vi "ni579x Host Align.vi"(0 "sync.resources":T1, 1 "sync.meas.Reference Clock":refnum<k21>, 2 "sync.meas.FPGA Clock x2":refnum<k21>, 3 "sync.meas.FPGA I/O":refnum<k21>) -> (4 "sync.resources":T1)   [LabVIEW 2015, in "ni579x Synchronization v1 FPGA.lvlib"]
doc: "*** THIS VI IS DEPRECATED. USE ni579x Host Align 2.vi ***\n\nAlign the targets participating in synchronization. This must occur before a signal can be synchronized.\n\nThere are two flavors of alignment to chose from -- Host Align and FPGA Align. The two flavors produce the same quality of synchronization, but differ in requirements and versatility of operation.\n\nWhen using <B>ni579x FPGA Align 2</B>, the Single Cycle Timed Loop (SCTL) rate (that this VI is in) must be an integer multiple of the <B>sync.cptr.Reference Clock</B> rate, and the SCTL clock must have a fixed phase relationship to the reference clock. Each target performs its alignment independently, so FPGA Align does not require a FPGA I/O line. It's also possible to use FPGA Align without host interaction. FPGA Align has 100% repeatability if-and-only-if the target-to-target phase relationship is low and does not change.\n\nWhen using <B>ni579x Host Align 2</B>, the SCTL rate may be arbitrary (yet still must have a fixed phase relationship to the other targets). The CPTR period may also be arbitrary. This alignment process is coordinated by the host, and requires an FPGA I/O line for orchestration. Host Align has 100% repeatability; if the hardware configuration remains constant, so will the level of synchronization.\n\n<B>Input Parameters</B>\n\n<B>sync.resources</B> identifies the Synchronization instance. 'sync.resources' is obtained from the ni579x Create VI of this library.\n\n<B>sync.meas.Reference Clock</B> is used by the measurement logic as the \"start\" signal. This is commonly PXI_Clk10.\n\n<B>sync.meas.FPGA Clock x2</B> is used by the measurement logic as the measurement clock. This clock must run at twice the rate of the FPGA Clock (the clock that drives the Single Cycle Timed Loop (SCTL) which this VI is in). This clock must also be derrived from the FPGA Clock, so that it has a fixed phase relationship. This is commonly IO Module\\Sample Clock x2.\n\n<B>sync.meas.FPGA I/O</B> is the FPGA I/O line that will be used to orchestrate starting the measurements. This is commonly a PXI Trig line.\n\nNote: For large NI chassis, make sure the PXI Trig line is routed to all bus segments that have targets participating in synchronization.\n\n<B>Output Parameters</B>\n\n<B>sync.resources</B> is the same instance that was passed in for 'sync.resources'."
uses:
  <instrlib>/ni579x/Synchronization/v1/FPGA/ni579x Synchronization v1 FPGA.lvlib
  <vilib>/eio/EIONode/EIONode.xnode
  <instrlib>/_niInstr/Basic Elements/v1/FPGA/niInstr Basic Elements v1 FPGA.lvlib
  <vilib>/rvi/LocalResourceManager/LocalResourceManager.xnode
  <vilib>/rvi/DataTransferAndStorage/Container/Common/niFpgaContainerGetUniqueNameForEmu.vi
  <vilib>/rvi/DataTransferAndStorage/Container/Common/niFpgaContainerSetEmuInfo.vi
  <vilib>/rvi/eio/common/nirviEmuReportErrorAndStop.vi
  <instrlib>/_niInstr/TDC/v1/FPGA/niInstr Overclocked TDC v1 FPGA.lvlib
  <vilib>/rvi/eio/common/nirviEmuTemplateMethod_errors.vi
  <instrlib>/ni579x/Synchronization/v1/FPGA/Implementation/Resources.ctl
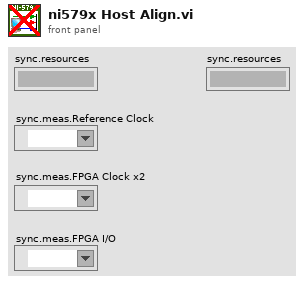
[diagram p1: front panel]
types:
  T1 = typedef "ni579x Synchronization v1 FPGA.lvlib/Resources.ctl" = cluster{"master":refnum<k21>, "meas.enable":refnum<k21>, "meas.ready":refnum<k21>, "meas.arm":refnum<k21>, "meas.valid":refnum<k21>, "meas.value":refnum<k21>, "meas.oversample clock":refnum<k21>, "meas.oversample factor":refnum<k21>, "cptr":refnum<k21>, "cptr.adjust":refnum<k21>, "cptr.period":refnum<k21>}
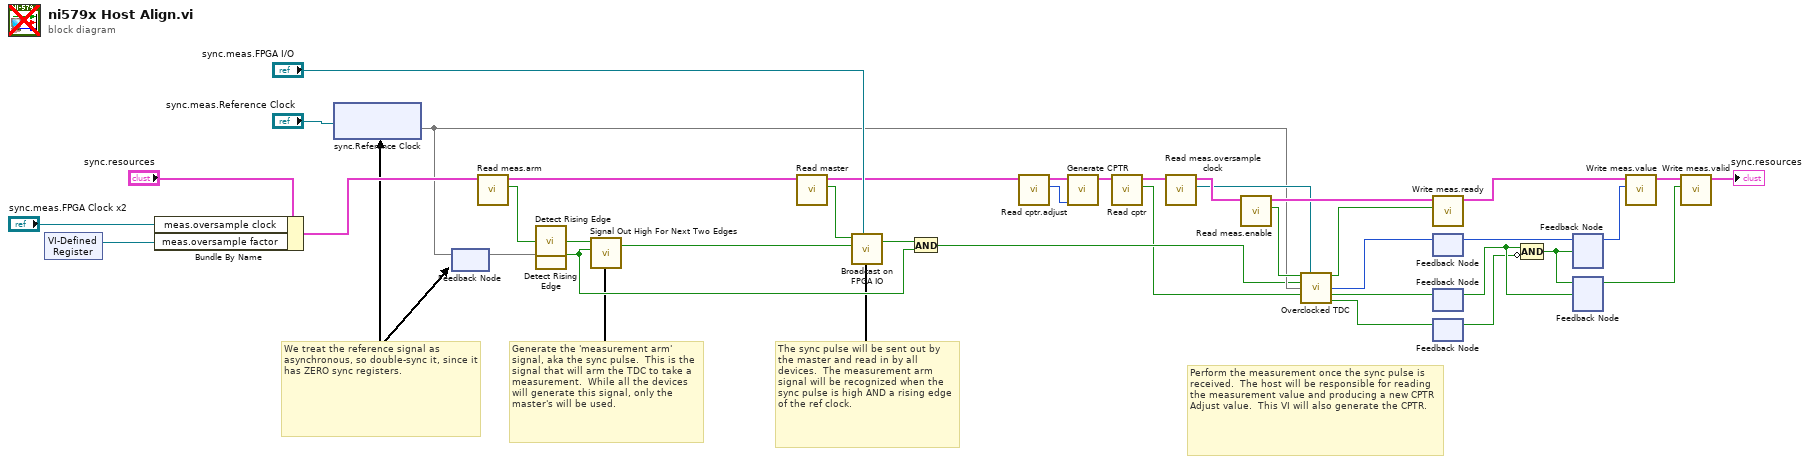
[diagram p0: block diagram]
diagram:
  # "We treat the reference signal as asynchronous, so double-sync it, since it has ZERO sync registers."
  # "Perform the measurement once the sync pulse is received.  The host will be responsible for reading the measurement value and producing a new CPTR Adjust value.  This VI will also generate the CPTR."
  # "The sync pulse will be sent out by the master and read in by all devices.  The measurement arm signal will be recognized when the sync pulse is high AND a rising edge of the ref clock."
  # "Generate the 'measurement arm' signal, aka the sync pulse.  This is the signal that will arm the TDC to take a measurement.  While all the devices will generate this signal, only the master's will be used."
  n1 = xnode "VI-Defined Register"() -> ("Register Out"=w18:refnum<k21>)
  n2 = Bundle By Name(cluster="sync.resources", "meas.oversample clock"="sync.meas.FPGA Clock x2", "meas.oversample factor"=w18) -> (w16:T1)
  n3 = xnode ("sync.Reference Clock")("FPGA I/O In"="sync.meas.Reference Clock") -> ("I/O Item"=w10)  [unwired: 1 out]
  n4 = feedback #1() -> (w36)  [unwired: 1 in]
  n5 = feedback-in #1(w10) -> ()
  n6 = call <instrlib>:"Read meas.arm.vi"("sync.resources"=w16) -> ("meas.arm"=w32:bool, "sync.resources"=w27:T1)  [unwired: 9 in]
  n7 = call <instrlib>:"Detect Rising Edge.vi"("signal"=w32) -> ("edge detected"=w37:bool)  [unwired: 14 in]
  n8 = call <instrlib>:"Detect Rising Edge.vi"("signal"=w36) -> ("edge detected"=w39:bool)  [unwired: 14 in]
  n9 = call <instrlib>:"Signal Out High For Next Two Edges.vi"("edge"=w39, "signal"=w37) -> ("signal for distribution"=w35:bool)  [unwired: 3 in]
  n10 = call <instrlib>:"Read master.vi"("sync.resources"=w27) -> ("master"=w31:bool, "sync.resources"=w24:T1)  [unwired: 9 in]
  n11 = call <instrlib>:"Broadcast on FPGA IO.vi"("FPGA I/O"="sync.meas.FPGA I/O", "signal in"=w35, "master"=w31) -> ("signal out"=w34:bool)  [unwired: 4 in]
  n12 = And(x=w34, y=w39) -> (x .and. y?=w9:bool)
  n13 = call <instrlib>:"Read cptr.adjust.vi"("sync.resources"=w24) -> ("cptr.adjust"=w23:u16, "sync.resources"=w25:T1)  [unwired: 9 in]
  n14 = call <instrlib>:"Generate CPTR.vi"("sync.cptr.adjust"=w23, "sync.resources"=w25) -> ("sync.resources"=w22:T1)  [unwired: 9 in]
  n15 = call <instrlib>:"Read cptr.vi"("sync.resources"=w22) -> ("cptr"=w8:bool, "sync.resources"=w20:T1)  [unwired: 9 in]
  n16 = call <instrlib>:"Read meas.oversample clock.vi"("sync.resources"=w20) -> ("meas.oversample clock"=w11:refnum<k21>, "sync.resources"=w15:T1)  [unwired: 9 in]
  n17 = call <instrlib>:"Read meas.enable.vi"("sync.resources"=w15) -> ("meas.enable"=w12:bool, "sync.resources"=w14:T1)  [unwired: 9 in]
  n18 = call <instrlib>:"Overclocked TDC.vi"("enable"=w12, "counter clock"=w11, "arm"=w9, "start"=w10, "stop"=w8) -> ("ready"=w6:bool, "count"=w7:u16, "count valid"=w5:bool, "rollover"=w4:bool)  [unwired: 6 in, 1 out]
  n19 = call <instrlib>:"Write meas.ready.vi"("meas.ready"=w6, "sync.resources"=w14) -> ("sync.resources"=w13:T1)  [unwired: 9 in]
  n20 = feedback #2() -> (w3:u16)  [unwired: 1 in]
  n21 = feedback-in #2(w7) -> ()
  n22 = feedback #3() -> (w2:bool)  [unwired: 1 in]
  n23 = feedback-in #3(w5) -> ()
  n24 = feedback #4() -> (w1:bool)  [unwired: 1 in]
  n25 = feedback-in #4(w4) -> ()
  n26 = Compound Arithmetic op=AND(w2, invert w1) -> (w30:bool)
  n27 = feedback #5() -> (w29:u16)  [unwired: 1 in]
  n28 = feedback-in #5(w3, w30) -> ()
  n29 = feedback #6() -> (w28:bool)  [unwired: 1 in]
  n30 = feedback-in #6(w30, w2) -> ()
  n31 = call <instrlib>:"Write meas.value.vi"("meas.value"=w29, "sync.resources"=w13) -> ("sync.resources"=w26:T1)  [unwired: 9 in]
  n32 = call <instrlib>:"Write meas.valid.vi"("meas.valid"=w28, "sync.resources"=w26) -> ("sync.resources"=→"sync.resources":T1)  [unwired: 9 in]
